vi "Event-MouseButton.vi"(8 "error in (no error)":errorcluster, 9 "MouseButtonEvent":T1, 10 "EventType":T4=enum."SDL_EVENT_WINDOW_DESTROYED", 11 "DVR Cluster In":T5={"CMD Queue"=refnum, "Config"={"Quit On Last Window Closed"=FALSE, "VSync"=enum."Disabled", "FPS Target"=30.0}, "Ctxt"={"VSync Enabled"=FALSE}, "Metrics"={"Uptime [ms]"=0, "Loop Time [ms]"=0, "Timer [ns]"=0, "Poll Events [ns]"=0, "Dequeue CMD [ns]"=0, "Update Layout [ns]"=0, "Render [ns]"=0}, "Debug"={"Unhandled Events"={}}, "ID To Window"={}, "Window To Handle"={}}) -> (0 "error out":errorcluster, 3 "DVR Cluster Out":T5={"CMD Queue"=refnum, "Config"={"Quit On Last Window Closed"=FALSE, "VSync"=enum."Disabled", "FPS Target"=30.0}, "Ctxt"={"VSync Enabled"=FALSE}, "Metrics"={"Uptime [ms]"=0, "Loop Time [ms]"=0, "Timer [ns]"=0, "Poll Events [ns]"=0, "Dequeue CMD [ns]"=0, "Update Layout [ns]"=0, "Render [ns]"=0}, "Debug"={"Unhandled Events"={}}, "ID To Window"={}, "Window To Handle"={}})   [LabVIEW 2020, in "GLF.lvlib" / "Engine.lvclass"]
uses:
  Engine.lvclass
  Engine.lvclass/Engine.ctl
  <vilib>/Utility/miscctls.llb/LVMapReplaceAction.ctl
  <vilib>/Saukko/LV SDL3/Sources/SDL3/Events/EventType--enum.ctl
  <vilib>/Saukko/LV SDL3/Sources/SDL3/Events/Events.lvlib
  Window/Window.lvclass
  VSync--enum.ctl
  Config--cluster.ctl
  Context--cluster.ctl
  Metrics--cluster.ctl
  Command--enum.ctl
  Command--cluster.ctl
  Command--queue.ctl
  <vilib>/Saukko/LV SDL3/Sources/SDL3/Video/WindowID--integer.ctl
  <vilib>/Saukko/LV SDL3/Sources/SDL3/Video/Video.lvlib
  DVR--cluster.ctl
  Debug--cluster.ctl
  <vilib>/Saukko/LV SDL3/Sources/SDL3/Mouse/MouseID--integer.ctl
  <vilib>/Saukko/LV SDL3/Sources/SDL3/Mouse/Mouse.lvlib
  <vilib>/Saukko/LV SDL3/Sources/SDL3/Events/MouseButtonEventData--cluster.ctl
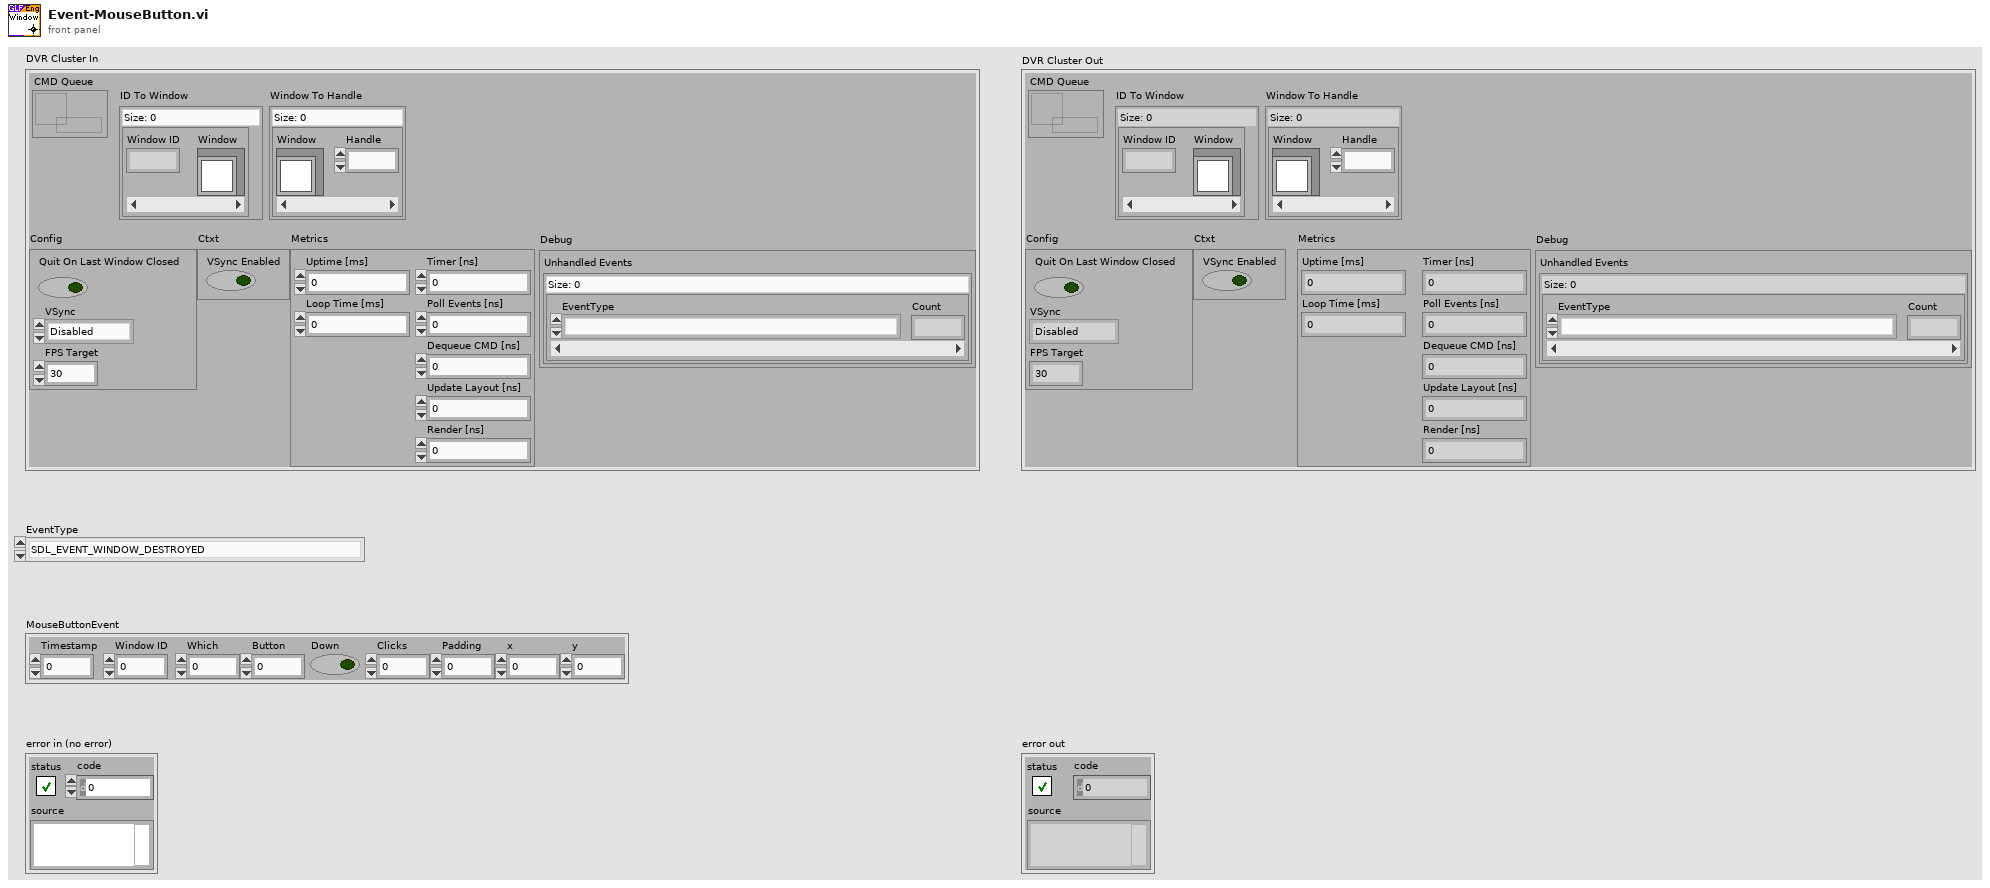
[diagram p1: front panel]
types:
  T1 = typedef "SDL3.lvlib/Events.lvlib/MouseButtonEventData--cluster.ctl" = cluster{"Timestamp":u64, "Window ID":T2, "Which":T3, "Button":u8, "Down":bool, "Clicks":u8, "Padding":u8, "x":sgl, "y":sgl}
  T2 = typedef "SDL3.lvlib/Video.lvlib/WindowID--integer.ctl" = u32
  T3 = typedef "SDL3.lvlib/Mouse.lvlib/MouseID--integer.ctl" = u32
  T4 = typedef "SDL3.lvlib/Events.lvlib/EventType--enum.ctl" = enum16{"LV_NONE", "LV_UNSUPPORTED", "SDL_EVENT_QUIT", "SDL_EVENT_LOCALE_CHANGED", "SDL_EVENT_SYSTEM_THEME_CHANGED", "SDL_EVENT_DISPLAY_ORIENTATION", "SDL_EVENT_DISPLAY_ADDED", "SDL_EVENT_DISPLAY_REMOVED", "SDL_EVENT_DISPLAY_MOVED", "SDL_EVENT_DISPLAY_DESKTOP_MODE_CHANGED", "SDL_EVENT_DISPLAY_CURRENT_MODE_CHANGED", "SDL_EVENT_DISPLAY_CONTENT_SCALE_CHANGED", "SDL_EVENT_WINDOW_SHOWN", "SDL_EVENT_WINDOW_HIDDEN", "SDL_EVENT_WINDOW_EXPOSED", "SDL_EVENT_WINDOW_MOVED", "SDL_EVENT_WINDOW_RESIZED", "SDL_EVENT_WINDOW_PIXEL_SIZE_CHANGED", "SDL_EVENT_WINDOW_METAL_VIEW_RESIZED", "SDL_EVENT_WINDOW_MINIMIZED", "SDL_EVENT_WINDOW_MAXIMIZED", "SDL_EVENT_WINDOW_RESTORED", "SDL_EVENT_WINDOW_MOUSE_ENTER", "SDL_EVENT_WINDOW_MOUSE_LEAVE", "SDL_EVENT_WINDOW_FOCUS_GAINED", "SDL_EVENT_WINDOW_FOCUS_LOST", "SDL_EVENT_WINDOW_CLOSE_REQUESTED", "SDL_EVENT_WINDOW_HIT_TEST", "SDL_EVENT_WINDOW_ICCPROF_CHANGED", "SDL_EVENT_WINDOW_DISPLAY_CHANGED", "SDL_EVENT_WINDOW_DISPLAY_SCALE_CHANGED", "SDL_EVENT_WINDOW_SAFE_AREA_CHANGED", "SDL_EVENT_WINDOW_OCCLUDED", "SDL_EVENT_WINDOW_ENTER_FULLSCREEN", "SDL_EVENT_WINDOW_LEAVE_FULLSCREEN", "SDL_EVENT_WINDOW_DESTROYED", "SDL_EVENT_WINDOW_HDR_STATE_CHANGED", "SDL_EVENT_KEY_DOWN", "SDL_EVENT_KEY_UP", "SDL_EVENT_TEXT_EDITING", "SDL_EVENT_TEXT_INPUT", "SDL_EVENT_KEYMAP_CHANGED", "SDL_EVENT_KEYBOARD_ADDED", "SDL_EVENT_KEYBOARD_REMOVED", "SDL_EVENT_TEXT_EDITING_CANDIDATES", "SDL_EVENT_MOUSE_MOTION", "SDL_EVENT_MOUSE_BUTTON_DOWN", "SDL_EVENT_MOUSE_BUTTON_UP", "SDL_EVENT_MOUSE_WHEEL", "SDL_EVENT_MOUSE_ADDED", "SDL_EVENT_MOUSE_REMOVED", "SDL_EVENT_JOYSTICK_AXIS_MOTION", "SDL_EVENT_JOYSTICK_BALL_MOTION", "SDL_EVENT_JOYSTICK_HAT_MOTION", "SDL_EVENT_JOYSTICK_BUTTON_DOWN", "SDL_EVENT_JOYSTICK_BUTTON_UP", "SDL_EVENT_JOYSTICK_ADDED", "SDL_EVENT_JOYSTICK_REMOVED", "SDL_EVENT_JOYSTICK_BATTERY_UPDATED", "SDL_EVENT_JOYSTICK_UPDATE_COMPLETE", "SDL_EVENT_GAMEPAD_AXIS_MOTION", "SDL_EVENT_GAMEPAD_BUTTON_DOWN", "SDL_EVENT_GAMEPAD_BUTTON_UP", "SDL_EVENT_GAMEPAD_ADDED", "SDL_EVENT_GAMEPAD_REMOVED", "SDL_EVENT_GAMEPAD_REMAPPED", "SDL_EVENT_GAMEPAD_TOUCHPAD_DOWN", "SDL_EVENT_GAMEPAD_TOUCHPAD_MOTION", "SDL_EVENT_GAMEPAD_TOUCHPAD_UP", "SDL_EVENT_GAMEPAD_SENSOR_UPDATE", "SDL_EVENT_GAMEPAD_UPDATE_COMPLETE", "SDL_EVENT_GAMEPAD_STEAM_HANDLE_UPDATED", "SDL_EVENT_FINGER_DOWN", "SDL_EVENT_FINGER_UP", "SDL_EVENT_FINGER_MOTION", "SDL_EVENT_CLIPBOARD_UPDATE", "SDL_EVENT_DROP_FILE", "SDL_EVENT_DROP_TEXT", "SDL_EVENT_DROP_BEGIN", "SDL_EVENT_DROP_COMPLETE", "SDL_EVENT_DROP_POSITION", "SDL_EVENT_AUDIO_DEVICE_ADDED", "SDL_EVENT_AUDIO_DEVICE_REMOVED", "SDL_EVENT_AUDIO_DEVICE_FORMAT_CHANGED", "SDL_EVENT_SENSOR_UPDATE", "SDL_EVENT_PEN_PROXIMITY_IN", "SDL_EVENT_PEN_PROXIMITY_OUT", "SDL_EVENT_PEN_DOWN", "SDL_EVENT_PEN_UP", "SDL_EVENT_PEN_BUTTON_DOWN", "SDL_EVENT_PEN_BUTTON_UP", "SDL_EVENT_PEN_MOTION", "SDL_EVENT_PEN_AXIS", "SDL_EVENT_CAMERA_DEVICE_ADDED", "SDL_EVENT_CAMERA_DEVICE_REMOVED", "SDL_EVENT_CAMERA_DEVICE_APPROVED", "SDL_EVENT_CAMERA_DEVICE_DENIED", "SDL_EVENT_RENDER_TARGETS_RESET", "SDL_EVENT_RENDER_DEVICE_RESET", "SDL_EVENT_POLL_SENTINEL", "SDL_EVENT_USER"}
  T5 = typedef "GLF.lvlib/Engine.lvclass/DVR--cluster.ctl" = cluster{"CMD Queue":T6, "Config":T7, "Ctxt":T9, "Metrics":T10, "Debug":T11, "ID To Window":map{T2, refnum<class "Window.lvclass">}, "Window To Handle":map{refnum<class "Window.lvclass">, i64}}
  T6 = typedef "GLF.lvlib/Engine.lvclass/Command--queue.ctl" = refnum<queue>
  T7 = typedef "GLF.lvlib/Engine.lvclass/Config--cluster.ctl" = cluster{"Quit On Last Window Closed":bool, "VSync":T8, "FPS Target":dbl}
  T8 = typedef "GLF.lvlib/Engine.lvclass/VSync--enum.ctl" = enum16{"Disabled", "Enabled", "Adaptative"}
  T9 = typedef "GLF.lvlib/Engine.lvclass/Context--cluster.ctl" = cluster{"VSync Enabled":bool}
  T10 = typedef "GLF.lvlib/Engine.lvclass/Metrics--cluster.ctl" = cluster{"Uptime [ms]":u64, "Loop Time [ms]":u64, "Timer [ns]":u64, "Poll Events [ns]":u64, "Dequeue CMD [ns]":u64, "Update Layout [ns]":u64, "Render [ns]":u64}
  T11 = typedef "GLF.lvlib/Engine.lvclass/Debug--cluster.ctl" = cluster{"Unhandled Events":map{T4, u64}}
  T12 = typedef "LVMapReplaceAction.ctl" = enum32{"Modify Entry only if found", "Add or Modify Entry", "Delete Entry"}
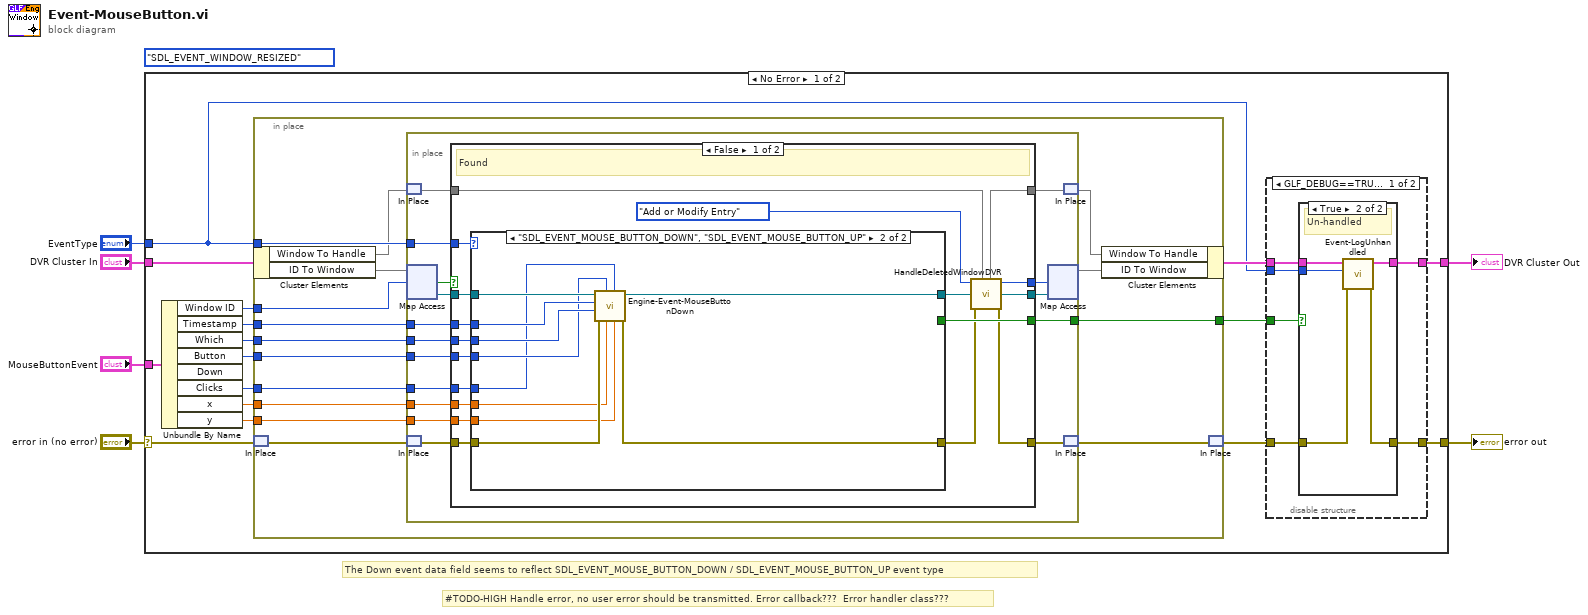
[diagram p0: block diagram]
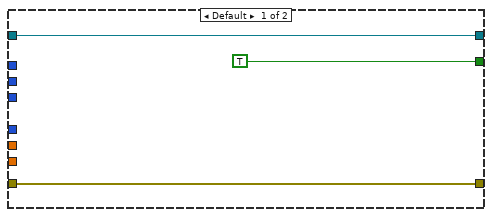
[diagram p2: hidden frame]
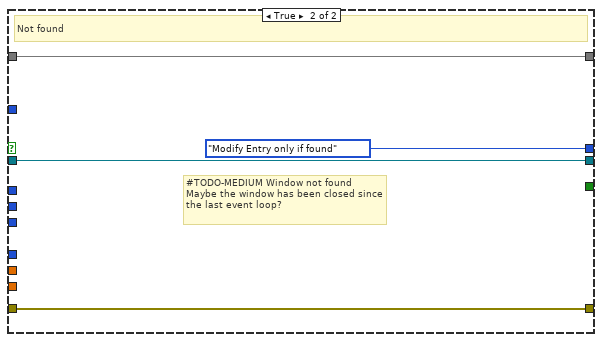
[diagram p3: hidden frame]
diagram:
  (unwired) EventType--enum."SDL_EVENT_WINDOW_RESIZED" ("EventType")
  # "The Down event data field seems to reflect SDL_EVENT_MOUSE_BUTTON_DOWN / SDL_EVENT_MOUSE_BUTTON_UP event type"
  # "#TODO-HIGH Handle error, no user error should be transmitted. Error callback???  Error handler class???"
  n1 = case shown="No Error" "error in (no error)" {
    selector: "error in (no error)" -> [w19 w104]
    tunnel: [w14 w104] -> w5
    tunnel: [w15 w103] -> w3
    tunnel: "DVR Cluster In" -> [w21 w103]
    tunnel: "MouseButtonEvent" -> [w22 _]
    tunnel: "EventType" -> [w13 _]
    frame No Error {
      n2 = Unbundle By Name(w22) -> ("Window ID"=w20:T2, "Timestamp"=w18:u64, "Which"=w11:T3, "Button"=w10:u8, "Clicks"=w9:u8, "x"=w8:sgl, "y"=w7:sgl)  [unwired: 1 out]
      n3 = in-place {
        in-place-border: w20 -> [w36]
        in-place-border: w18 -> [w33]
        in-place-border: w13 -> [w31]
        in-place-border: [w30] -> w12
        in-place-border: w11 -> [w29]
        in-place-border: w10 -> [w28]
        in-place-border: w9 -> [w25]
        in-place-border: w8 -> [w24]
        in-place-border: w7 -> [w23]
        n4 = in-place-cluster #1(w21) -> ("Window To Handle"=w27:map{refnum<class "Window.lvclass">, i64}, "ID To Window"=w37:map{T2, refnum<class "Window.lvclass">})
        n5 = in-place-match #2(w19) -> (w35:errorcluster)
        n6 = in-place {
          in-place-border: w33 -> [w47]
          in-place-border: w31 -> [w46]
          in-place-border: [w45] -> w30
          in-place-border: w29 -> [w44]
          in-place-border: w28 -> [w43]
          in-place-border: w25 -> [w40]
          in-place-border: w24 -> [w39]
          in-place-border: w23 -> [w38]
          n7 = in-place-match #3(w27) -> (w42:map{refnum<class "Window.lvclass">, i64})
          n8 = in-place-map #4(w37, w36) -> (w52:refnum<class "Window.lvclass">, w53:bool)  [unwired: 1 in]
          n9 = in-place-match #5(w35) -> (w50:errorcluster)
          n10 = case shown="False" w53 {
            tunnel: w52 -> [w70 w85]
            tunnel: [w60 LVMapReplaceAction."Modify Entry only if found" ("Replace Action")] -> w51
            tunnel: [w64 w86] -> w49
            tunnel: w50 -> [w69 w86]
            tunnel: [w59 w85] -> w48
            tunnel: w47 -> [w68 _]
            tunnel: w46 -> [w67 _]
            tunnel: [w66 _] -> w45
            tunnel: w44 -> [w63 _]
            tunnel: w43 -> [w62 _]
            tunnel: w42 -> [w54 w84]
            tunnel: [w61 w84] -> w41
            tunnel: w40 -> [w57 _]
            tunnel: w39 -> [w56 _]
            tunnel: w38 -> [w55 _]
            frame False {
              # "Found"
              n11 = case shown="\"SDL_EVENT_MOUSE_BUTTON_DOWN\", \"SDL_EVENT_MOUSE_BUTTON_UP\"" w67 {
                tunnel: [w71 w83] -> w65
                tunnel: [w72 w82] -> w59
                tunnel: w70 -> [w72 w81]
                tunnel: w69 -> [w71 w80]
                tunnel: w68 -> [_ w79]
                tunnel: [TRUE _] -> w66
                tunnel: w63 -> [_ w78]
                tunnel: w62 -> [_ w77]
                tunnel: w57 -> [_ w76]
                tunnel: w56 -> [_ w75]
                tunnel: w55 -> [_ w74]
                frame Default {
                }
                frame "SDL_EVENT_MOUSE_BUTTON_DOWN", "SDL_EVENT_MOUSE_BUTTON_UP" {
                  n12 = call "Engine-Event-MouseButtonDown.vi"("y"=w74, "Clicks"=w76, "x"=w75, "Button"=w77, "error in (no error)"=w80, "Which"=w78, "Timestamp"=w79, "GLF Window in"=w81) -> ("error out"=w83:errorcluster, "GLF Window out"=w82:refnum<class "Window.lvclass">)  [unwired: 2 in]
                }
              }
              n13 = call "HandleDeletedWindowDVR.vi"("Window To Handle In"=w54, "error in (no error)"=w65, "Window"=w59, "Replace Action In"=LVMapReplaceAction."Add or Modify Entry" ("Replace Action")) -> ("error out"=w64:errorcluster, "Replace Action Out"=w60:T12, "Window To Handle Out"=w61:map{refnum<class "Window.lvclass">, i64})  [unwired: 5 in]
            }
            frame True {
              # "#TODO-MEDIUM Window not found\nMaybe the window has been closed since the last event loop?"
              # "Not found"
            }
          }
          n14 = in-place-map #4(w48, w51) -> (w32:map{T2, refnum<class "Window.lvclass">})  [unwired: 2 out]
          n15 = in-place-match #3(w41) -> (w26:map{refnum<class "Window.lvclass">, i64})
          n16 = in-place-match #5(w49) -> (w34:errorcluster)
        }
        n17 = in-place-cluster #1("Window To Handle"=w26, "ID To Window"=w32) -> (w16:T5)
        n18 = in-place-match #2(w34) -> (w17:errorcluster)
      }
      n19 = disable-structure shown="GLF_DEBUG==TRUE" {
        disable-tunnel: w17 -> [w93 w101]
        disable-tunnel: w16 -> [w92 w102]
        disable-tunnel: [w91 w102] -> w15
        disable-tunnel: [w90 w101] -> w14
        disable-tunnel: w13 -> [w89 _]
        disable-tunnel: w12 -> [w88 _]
        frame condition #0 (active) {
          n20 = case shown="True" w88 {
            tunnel: w93 -> [w94 w100]
            tunnel: w92 -> [w95 w99]
            tunnel: [w95 w98] -> w91
            tunnel: [w94 w97] -> w90
            tunnel: w89 -> [_ w96]
            frame False {
              # "Handled"
            }
            frame True {
              # "Un-handled"
              n21 = call "Event-LogUnhandled.vi"("error in (no error)"=w100, "EventType"=w96, "DVR Cluster In"=w99) -> ("error out"=w97:errorcluster, "DVR Cluster Out"=w98:T5)  [unwired: 7 in]
            }
          }
        }
        frame condition #1 {
        }
      }
    }
    frame Error {
    }
  }
  "error out" <- w5
  "DVR Cluster Out" <- w3
